vi "Obtain Doc Title.vi"(8 "error in (no error)":errorcluster, 11 "LV DEV in":refnum<class "LV DEV.lvclass">) -> (0 "error out":errorcluster, 3 "LV DEV out":refnum<class "LV DEV.lvclass">)   [LabVIEW 2016, in "LV DEV.lvclass"]
uses:
  LV DEV.lvclass
  D:/MDI Project/source code/Document/LV Doc/LV Doc.lvclass
  D:/MDI Project/source code/Document/Document base/Document.lvclass
  LV Doc.lvclass/LV Doc.ctl
  Document base/Document.lvclass/Document.ctl
  property/Read VI Reference.vi
  Document base/property/Write Doc Title.vi
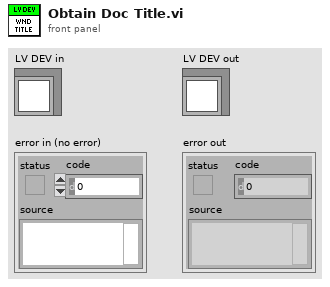
[diagram p1: front panel]
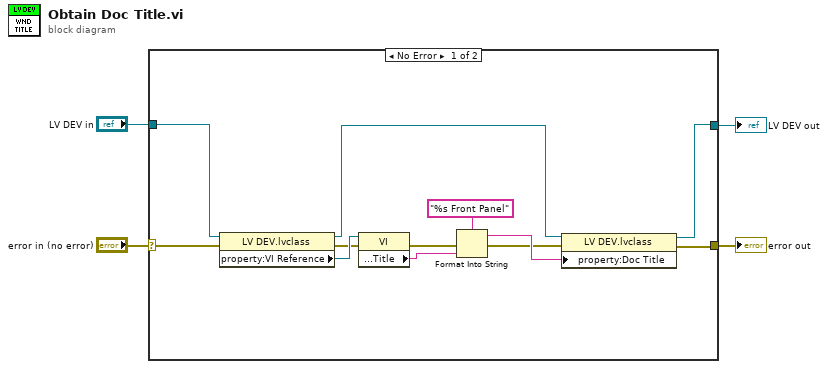
[diagram p0: block diagram]
diagram:
  n1 = case shown="No Error" "error in (no error)" {
    selector: "error in (no error)" -> [w13 w17]
    tunnel: [w6 w17] -> w3
    tunnel: [w7 w18] -> w1
    tunnel: "LV DEV in" -> [w8 w18]
    frame No Error {
      n2 = property class="LV DEV.lvclass"(reference=w8, error in=w13) -> (reference out=w5:refnum<class "LV DEV.lvclass">, error out=w11:errorcluster, "property:VI Reference"=w12:refnum<vi>)
      n3 = property class="VI"(reference=w12, error in=w11) -> (error out=w15:errorcluster, "Front Panel.Title"=w14:string)  [unwired: 1 out]
      n4 = Format Into String(format string="%s Front Panel", error in=w15, w14) -> (resulting string=w10:string, error out=w9:errorcluster)  [unwired: 1 in]
      n5 = property class="LV DEV.lvclass"(reference=w5, error in=w9, "property:Doc Title"=w10) -> (reference out=w7:refnum<class "LV DEV.lvclass">, error out=w6:errorcluster)
    }
    frame Error {
    }
  }
  "error out" <- w3
  "LV DEV out" <- w1
